vi "HaloControllerWithDeadband.vi"(0 "Throttle":dbl, 5 "Wheel":dbl, 7 "Deadband+":dbl=0.15, 9 "Sensitivity":dbl=0.7, 11 "QuikTurnButton":bool) -> (4 "Left Output":dbl, 6 "Right Output":dbl)   [LabVIEW 2016]
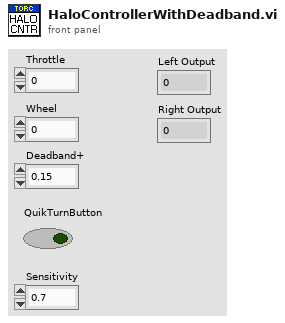
[diagram p1: front panel]
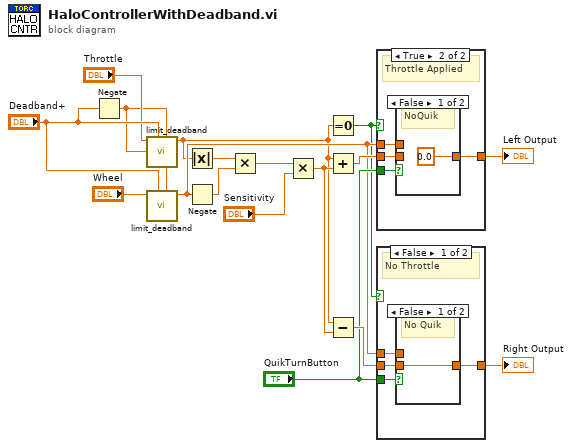
[diagram p0: block diagram]
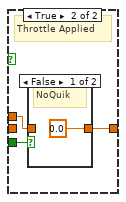
[diagram p3: hidden frame]
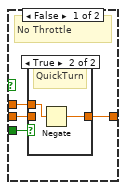
[diagram p5: hidden frame]
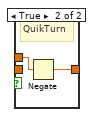
[diagram p7: hidden frame]
diagram:
  n1 = Negate(x="Deadband+") -> (-x=w3:dbl)
  n2 = call "limit_deadband.vi"("lower limit"=w3, "upper limit"="Deadband+", "Val"="Throttle") -> ("Val Out"=w2:dbl)  [unwired: 8 in]
  n3 = call "limit_deadband.vi"("lower limit"=w3, "upper limit"="Deadband+", "Val"="Wheel") -> ("Val Out"=w4:dbl)  [unwired: 8 in]
  n4 = Absolute Value(x=w2) -> (abs(x)=w17:dbl)
  n5 = Negate(x=w4) -> (-x=w14:dbl)
  n6 = Multiply(x=w17, y=w14) -> (x*y=w16:dbl)
  n7 = Multiply(x=w16, y="Sensitivity") -> (x*y=w15:dbl)
  n8 = Equal To 0?(x=w2) -> (x = 0?=w1:bool)
  n9 = Add(x=w2, y=w15) -> (x+y=w9:dbl)
  n10 = Subtract(x=w2, y=w15) -> (x-y=w10:dbl)
  n11 = case shown="True" w1 {
    tunnel: w9 -> [w20 w26]
    tunnel: [w21 w27] -> w13
    tunnel: w4 -> [w19 w28]
    tunnel: "QuikTurnButton" -> [w18 w25]
    frame False {
      # "No Throttle"
      n12 = case shown="True" w18 {
        tunnel: w20 -> [w22 _]
        tunnel: [w22 w23] -> w21
        tunnel: w19 -> [_ w24]
        frame False {
        }
        frame True {
          # "QuickTurn"
          n13 = Negate(x=w24) -> (-x=w23:dbl)
        }
      }
    }
    frame True {
      # "Throttle Applied"
      n14 = case shown="False" w25 {
        tunnel: w28 -> [_ w31]
        tunnel: [0.0 w30] -> w27
        tunnel: w26 -> [_ _]
        frame False {
          # "NoQuik"
        }
        frame True {
          # "QuikTurn"
          n15 = Negate(x=w31) -> (-x=w30:dbl)
        }
      }
    }
  }
  "Left Output" <- w13
  n16 = case shown="False" w1 {
    tunnel: [w35 w40] -> w12
    tunnel: w10 -> [w34 _]
    tunnel: w4 -> [w33 w39]
    tunnel: "QuikTurnButton" -> [w32 w38]
    frame False {
      # "No Throttle"
      n17 = case shown="False" w32 {
        tunnel: w34 -> [w36 _]
        tunnel: [w36 w37] -> w35
        tunnel: w33 -> [_ w37]
        frame False {
          # "No Quik"
        }
        frame True {
          # "QuickTurn"
        }
      }
    }
    frame True {
      # "Throttle Applied"
      n18 = case shown="False" w38 {
        tunnel: [0.0 w42] -> w40
        tunnel: w39 -> [_ w42]
        frame False {
          # "NoQuik"
        }
        frame True {
          # "QuikTurn"
        }
      }
    }
  }
  "Right Output" <- w12
